vi "copy alarmList database.vi"(8 "error in (no error)":errorcluster) -> (0 "error out":errorcluster)   [LabVIEW 2016]
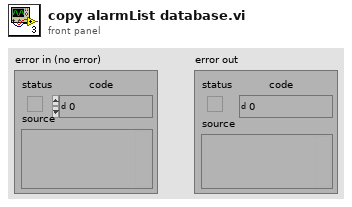
[diagram p1: front panel]
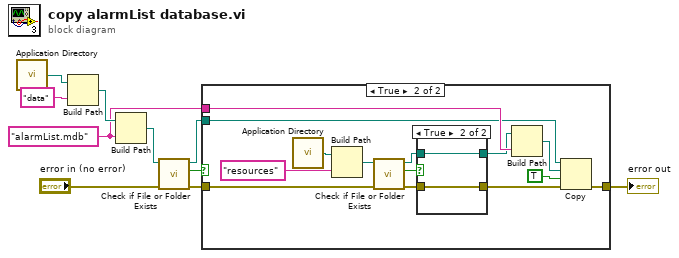
[diagram p0: block diagram]
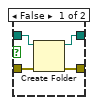
[diagram p3: hidden frame]
diagram:
  w7 = "alarmList.mdb" ("名称或相对路径")
  n1 = call <vilib>:"Application Directory.vi"() -> ("Application Directory"=w10:path)
  n2 = Build Path(base path=w10, name or relative path="data" ("名称或相对路径")) -> (appended path=w8:path)
  n3 = Build Path(base path=w8, name or relative path=w7) -> (appended path=w6:path)
  n4 = call <vilib>:"Check if File or Folder Exists.vi"("error in (no error)"="error in (no error)", "path"=w6) -> ("error out"=w3:errorcluster, "file or folder exists?"=w4:bool, "dup path"=w5:path)  [unwired: 7 in]
  n5 = case shown="True" w4 {
    tunnel: w7 -> [_ w22]
    tunnel: w5 -> [_ w13]
    tunnel: w3 -> [_ w12]
    tunnel: [_ w11] -> w1
    frame False {
    }
    frame True {
      n6 = call <vilib>:"Application Directory.vi"() -> ("Application Directory"=w23:path)
      n7 = Build Path(base path=w23, name or relative path="resources" ("名称或相对路径")) -> (appended path=w21:path)
      n8 = call <vilib>:"Check if File or Folder Exists.vi"("error in (no error)"=w12, "path"=w21) -> ("error out"=w19:errorcluster, "file or folder exists?"=w18:bool, "dup path"=w20:path)  [unwired: 7 in]
      n9 = case shown="True" w18 {
        tunnel: w20 -> [w28 w30]
        tunnel: w19 -> [w27 w29]
        tunnel: [w26 w30] -> w17
        tunnel: [w25 w29] -> w14
        frame False {
          n10 = Create Folder(path (use dialog)=w28, error in=w27) -> (created path=w26:path, error out=w25:errorcluster)  [unwired: 1 in, 1 out]
        }
        frame True {
        }
      }
      n11 = Build Path(base path=w17, name or relative path=w22) -> (appended path=w16:path)
      n12 = Copy(8:w14, 9:TRUE ("覆盖(F)"), 10:w16, 11:w13) -> (0:w11:errorcluster)  [unwired: 1 in, 2 out]
    }
  }
  "error out" <- w1
